vi "CreateMeasureRangeNode.vi"(7 "DOM Document":refnum<k20>, 8 "Error In":errorcluster, 10 "Range Function":enum16{"Voltage", "Current"}(ring), 11 "Measure Configuration":T1={"Enabled?"=FALSE, "Count"=1, "Interval (sec)"=0.025, "Voltage Auto Range Enabled?"=TRUE, "Voltage High Limit (V or A)"=0.0, "Voltage Low Limit (V or A)"=0.0, "Current Auto Range Enabled?"=TRUE, "Current High Limit (V or A)"=0.0, "Current Low Limit (V or A)"=0.0} {"Count" min=1 step=1}) -> (0 "Error Out":errorcluster, 3 "Range Node":refnum<k20>)   [LabVIEW 2013]
uses:
  MeasureConfiguration.ctl
  libs/LV-Utilities/LV-Utilities.lvlib
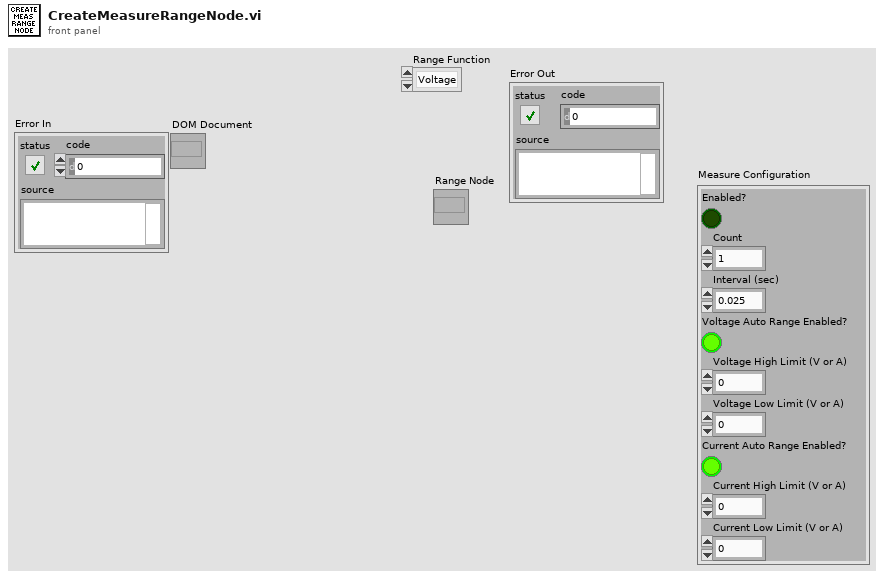
[diagram p1: front panel]
types:
  T1 = typedef "MeasureConfiguration.ctl" = cluster{"Enabled?":bool, "Count":u8, "Interval (sec)":dbl, "Voltage Auto Range Enabled?":bool, "Voltage High Limit (V or A)":dbl, "Voltage Low Limit (V or A)":dbl, "Current Auto Range Enabled?":bool, "Current High Limit (V or A)":dbl, "Current Low Limit (V or A)":dbl}
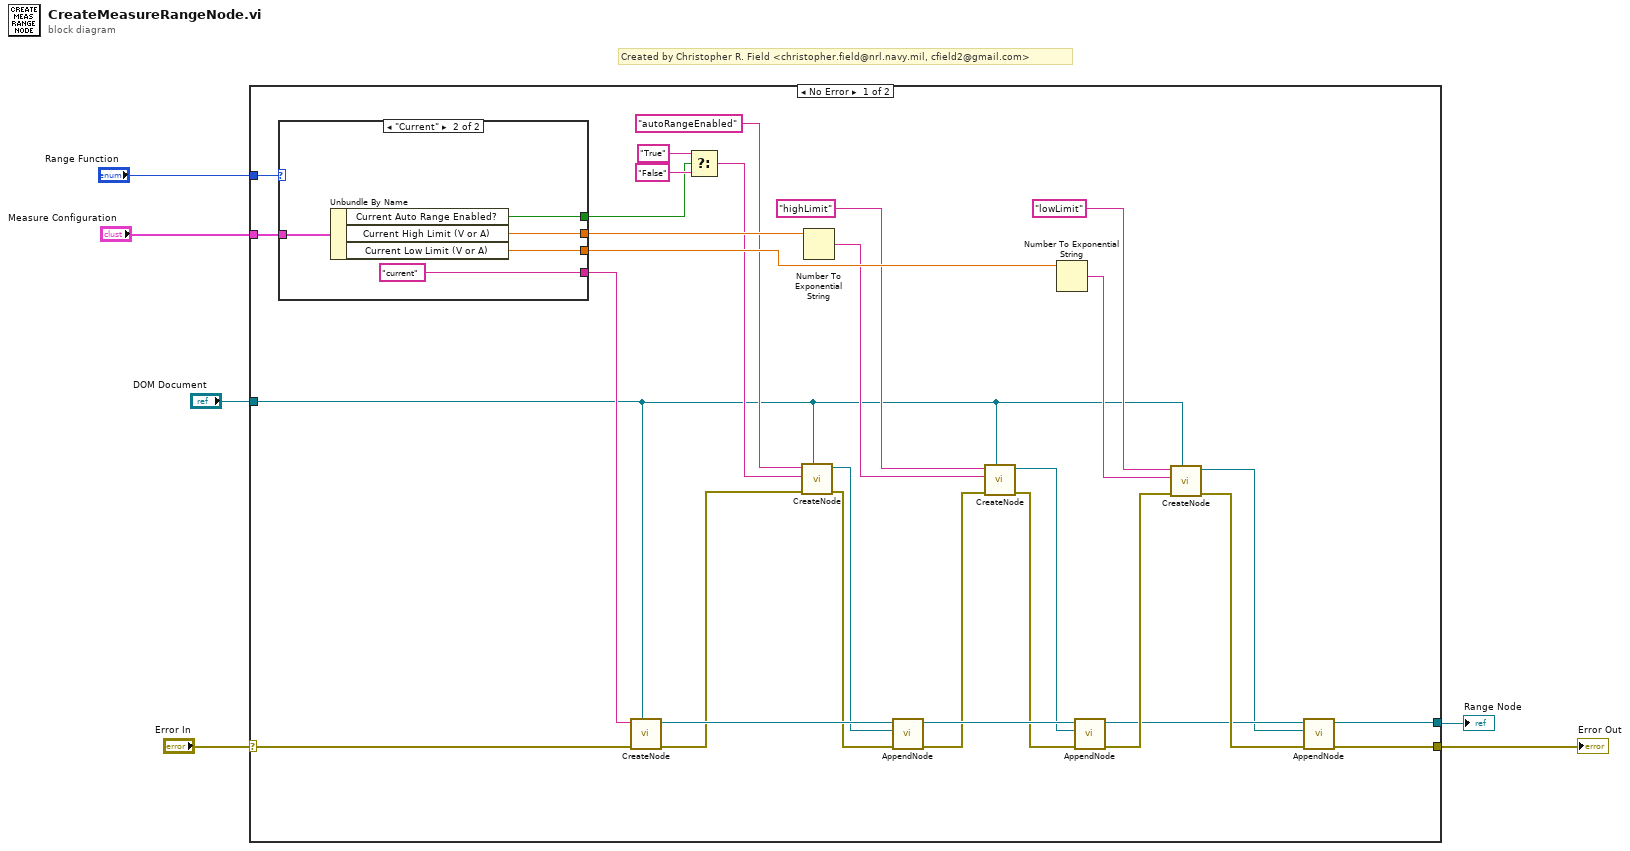
[diagram p0: block diagram]
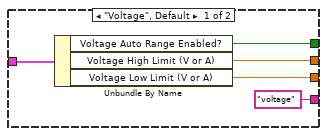
[diagram p2: hidden frame]
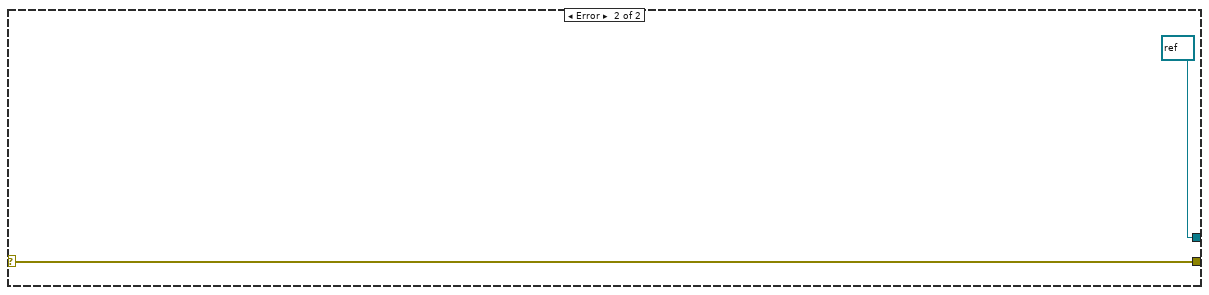
[diagram p3: hidden frame]
diagram:
  # "Created by Christopher R. Field <christopher.field@nrl.navy.mil, cfield2@gmail.com>"
  n1 = case shown="No Error" "Error In" {
    selector: "Error In" -> [w29 w48]
    tunnel: "DOM Document" -> [w21 _]
    tunnel: [w18 refnum<k20> refnum ("Wirings Node 2")] -> w4
    tunnel: [w19 w48] -> w3
    tunnel: "Measure Configuration" -> [w34 _]
    tunnel: "Range Function" -> [w33 _]
    frame No Error {
      n2 = case shown="\"Current\"" w33 {
        tunnel: w34 -> [w41 w46]
        tunnel: ["voltage" ("Tag Name") "current" ("Tag Name")] -> w28
        tunnel: [w39 w44] -> w32
        tunnel: [w38 w43] -> w31
        tunnel: [w37 w42] -> w30
        frame "Voltage", Default {
          n3 = Unbundle By Name(w41) -> ("Voltage Auto Range Enabled?"=w39:bool, "Voltage High Limit (V or A)"=w38:dbl, "Voltage Low Limit (V or A)"=w37:dbl)
        }
        frame "Current" {
          n4 = Unbundle By Name(w46) -> ("Current Auto Range Enabled?"=w44:bool, "Current High Limit (V or A)"=w43:dbl, "Current Low Limit (V or A)"=w42:dbl)
        }
      }
      n5 = call "CreateNode.vi"("DOM Document"=w21, "Error In"=w29, "Tag Name"=w28) -> ("Error out"=w10:errorcluster, "Node"=w14:refnum<k20>)  [unwired: 7 in]
      n6 = Select(t="True", s=w32, f="False") -> (s? t:f=w26:string)
      n7 = call "CreateNode.vi"("DOM Document"=w21, "Error In"=w10, "Text"=w26, "Tag Name"="autoRangeEnabled") -> ("Error out"=w11:errorcluster, "Node"=w9:refnum<k20>)  [unwired: 6 in]
      n8 = Number To Exponential String(number=w31) -> (E-format string=w25:string)  [unwired: 3 in]
      n9 = call "AppendNode.vi"("Error In"=w11, "Child Node"=w9, "Parent Node In"=w14) -> ("Error Out"=w12:errorcluster, "Parent Node Out"=w15:refnum<k20>)  [unwired: 7 in]
      n10 = call "CreateNode.vi"("DOM Document"=w21, "Error In"=w12, "Text"=w25, "Tag Name"="highLimit") -> ("Error out"=w13:errorcluster, "Node"=w8:refnum<k20>)  [unwired: 6 in]
      n11 = Number To Exponential String(number=w30) -> (E-format string=w22:string)  [unwired: 3 in]
      n12 = call "AppendNode.vi"("Error In"=w13, "Child Node"=w8, "Parent Node In"=w15) -> ("Error Out"=w17:errorcluster, "Parent Node Out"=w16:refnum<k20>)  [unwired: 7 in]
      n13 = call "CreateNode.vi"("DOM Document"=w21, "Error In"=w17, "Text"=w22, "Tag Name"="lowLimit") -> ("Error out"=w20:errorcluster, "Node"=w7:refnum<k20>)  [unwired: 6 in]
      n14 = call "AppendNode.vi"("Error In"=w20, "Child Node"=w7, "Parent Node In"=w16) -> ("Error Out"=w19:errorcluster, "Parent Node Out"=w18:refnum<k20>)  [unwired: 7 in]
    }
    frame Error {
    }
  }
  "Range Node" <- w4
  "Error Out" <- w3
